vi "GetSystemInfo.vi"(8 "error in (no error)":errorcluster) -> (0 "error out":errorcluster, 2 "Screen Y/2":i32, 3 "Screen X/2":i32, 4 "Screen Y":i32, 6 "Screen X":i32)   [LabVIEW 2015]
uses:
  User32.dll
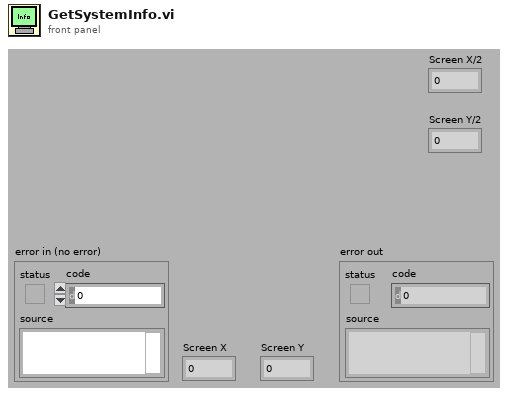
[diagram p1: front panel]
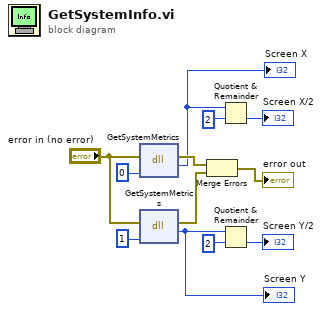
[diagram p0: block diagram]
diagram:
  n1 = dll-call lib="User32.dll" fn="GetSystemMetrics"(error in="error in (no error)", "nIndex"=0) -> (error out=w9:errorcluster, "WINAPI"=w6:i32)  [unwired: 3 in, 1 out]
  "Screen X" <- w6
  n2 = dll-call lib="User32.dll" fn="GetSystemMetrics"(error in="error in (no error)", "nIndex"=1) -> (error out=w8:errorcluster, "WINAPI"=w2:i32)  [unwired: 3 in, 1 out]
  "Screen Y" <- w2
  n3 = Merge Errors(w9, w8) -> (→"error out":errorcluster)
  n4 = Quotient & Remainder(x=w6, y=2) -> (floor(x/y)=→"Screen X/2":i32)  [unwired: 1 out]
  n5 = Quotient & Remainder(x=w2, y=2) -> (floor(x/y)=→"Screen Y/2":i32)  [unwired: 1 out]
